vi "Set File Paths.vi"(8 "error in (no error)":errorcluster, 9 "Paths":path[](array[path]), 10 "Path [use Paths]":path, 11 "Carya Config in":refnum<class "Carya Config.lvclass">) -> (0 "error out":errorcluster, 3 "Carya Config out":refnum<class "Carya Config.lvclass">)   [LabVIEW 2013, in "Carya Config.lvclass"]
doc: "Copyright 2018, Carya Automatisering, Wiebe Walstra."
uses:
  Carya Config.lvclass
  Carya Config.lvclass/Carya Config.ctl
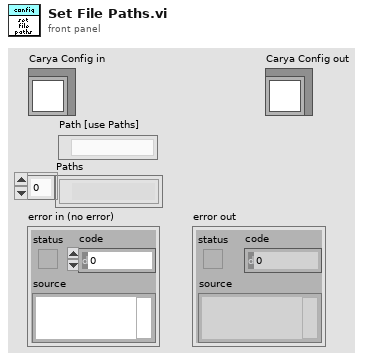
[diagram p1: front panel]
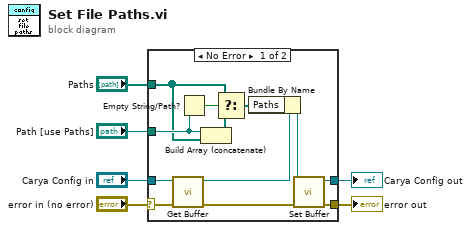
[diagram p0: block diagram]
diagram:
  n1 = case shown="No Error" "error in (no error)" {
    selector: "error in (no error)" -> [w18 w20]
    tunnel: [w15 w20] -> w5
    tunnel: [w14 w19] -> w3
    tunnel: "Carya Config in" -> [w16 w19]
    tunnel: "Path [use Paths]" -> [w12 _]
    tunnel: "Paths" -> [w10 _]
    frame No Error {
      n2 = call-dynamic "Get Buffer.vi"("error in (no error)"=w18, "Carya Config in"=w16) -> ("error out"=w17:errorcluster, "Config"=w8:refnum<class "Carya Config.lvclass">)  [unwired: 8 in]
      n3 = Empty String/Path?(string/path=w12) -> (empty?=w13:bool)
      n4 = Build Array (concatenate)(w12, w10) -> (w11:path[])
      n5 = Select(t=w10, s=w13, f=w11) -> (s? t:f=w9:path[])
      n6 = Bundle By Name(cluster=w8, "Paths"=w9) -> (w7:refnum<class "Carya Config.lvclass">)
      n7 = call-dynamic "Set Buffer.vi"("error in (no error)"=w17, "Carya Config"=w7) -> ("error out"=w15:errorcluster, "Carya Config out"=w14:refnum<class "Carya Config.lvclass">)  [unwired: 8 in]
    }
    frame Error {
    }
  }
  "error out" <- w5
  "Carya Config out" <- w3
